vi "Convert Enum.vi"(10 "Transport":refnum<class "Transport.lvclass">) -> (2 "Actor Type":T1)   [LabVIEW 2025, in "jettl.lvlib" / "Actor.lvlib"]
uses:
  Actor.lvlib
  Actor Type.ctl
  Transport/Queue/Queue.lvlib
  Transport/Event/Event.lvlib
  Transport/Notifier/Notifier.lvlib
  Transport/Transport/Transport.lvclass
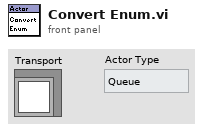
[diagram p1: front panel]
types:
  T1 = typedef "jettl.lvlib/Actor.lvlib/Actor Type.ctl" = enum16{"Queue", "Event", "Notifier"}
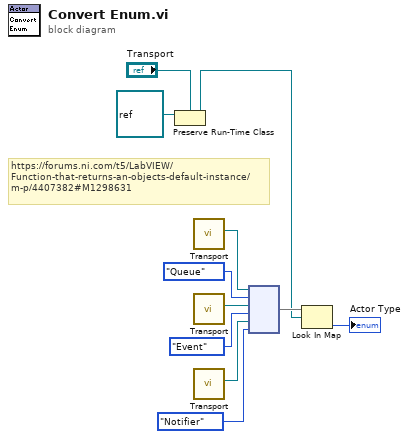
[diagram p0: block diagram]
diagram:
  # "https://forums.ni.com/t5/LabVIEW/Function-that-returns-an-objects-default-instance/m-p/4407382#M1298631"
  n1 = Preserve Run-Time Class(object in=refnum<class> refnum ("LabVIEW Object"), 2:"Transport") -> (object out=w2:refnum<class "Transport.lvclass">)  [unwired: 1 in, 1 out]
  n2 = call "Transport.vi"() -> ("Transport"=w11:refnum<class "Transport.lvclass">)  [unwired: 11 in]
  n3 = call "Transport.vi"() -> ("Transport"=w9:refnum<class "Transport.lvclass">)  [unwired: 11 in]
  n4 = call "Transport.vi"() -> ("Transport"=w8:refnum<class "Transport.lvclass">)  [unwired: 11 in]
  n5 = node(w11, Actor_Type."Queue" ("Actor Type"), w9, Actor_Type."Event" ("Actor Type"), w8, Actor_Type."Notifier" ("Actor Type")) -> (w5:map{refnum<class "Transport.lvclass">, T1})
  n6 = Look In Map(map=w5, key=w2) -> (value=→"Actor Type":T1)  [unwired: 1 in, 1 out]
